vi "fom_parser.vi"(1 "fom_path (in)":path=path "C:/data/projects/730 - Engineering Laboratory/04 - Smart Grid/HLA Based Code Autogeneration/support/fom_examples/FedManager.xml", 5 "error in (no error)":errorcluster) -> (15 "interaction_descriptors (out)":T1[](array[typedef]), 19 "error out":errorcluster)   [LabVIEW 2016]
uses:
  pre-build/support/controls/raw_object_interaction_descriptor.ctl
  <vilib>/xml/Load XML File.vi
  <vilib>/xml/Close Reference(Node).vi
  <vilib>/xml/NI_XML.lvlib
  <resource>/objmgr/DOMUserDefRef.rc
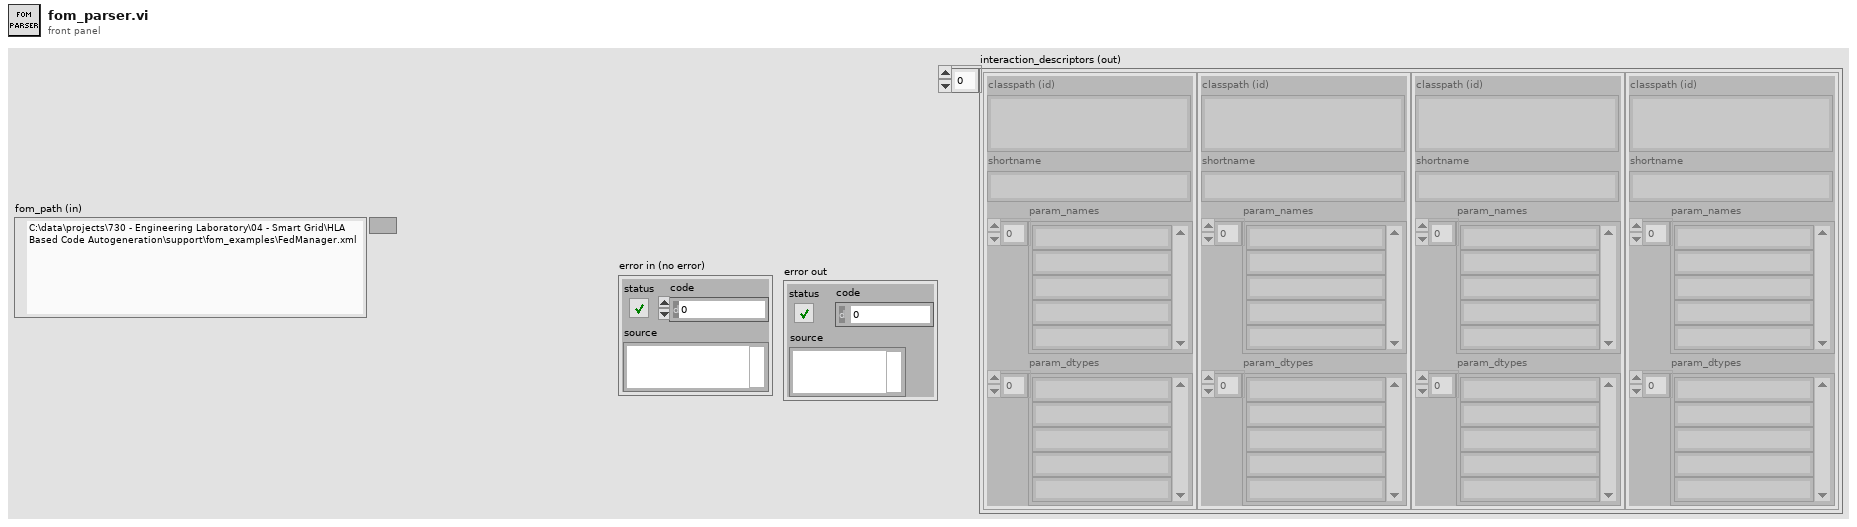
[diagram p1: front panel]
types:
  T1 = typedef "raw_object_interaction_descriptor.ctl" = cluster{"classpath (id)":string, "shortname":string, "param_names":string[], "param_dtypes":string[]}
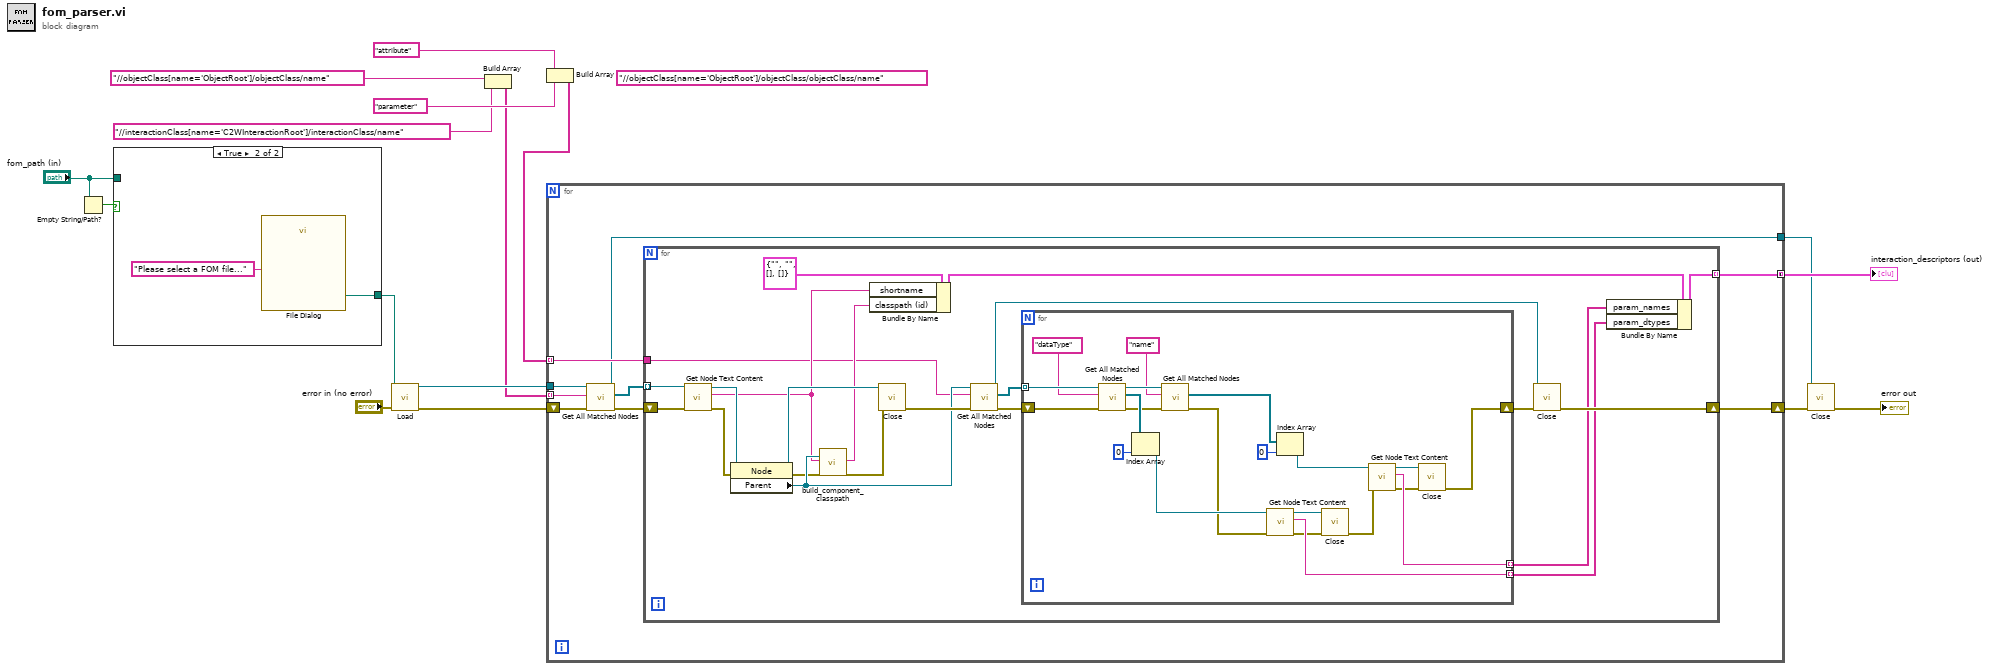
[diagram p0: block diagram]
diagram:
  (unwired) "//objectClass[name='ObjectRoot']/objectClass/objectClass/name"
  n1 = Empty String/Path?(string/path="fom_path (in)") -> (empty?=w12:bool)
  n2 = case shown="True" w12 {
    tunnel: [w17 w18] -> w10
    tunnel: "fom_path (in)" -> [w17 _]
    frame False {
    }
    frame True {
      n3 = call "File Dialog"("prompt"="Please select a FOM file...") -> ("selected path"=w18:path)  [unwired: 11 in, 3 out]
    }
  }
  n4 = call-poly <vilib>:"Load.vi"("path to XML document"=w10, "error in (no error)"="error in (no error)") -> ("DOM document out"=w16:refnum<k20>, "error out"=w15:errorcluster)  [unwired: 11 in, 1 out]
  n5 = Build Array("//objectClass[name='ObjectRoot']/objectClass/name", "//interactionClass[name='C2WInteractionRoot']/interactionClass/name") -> (w5:string[])
  n6 = Build Array("attribute", "parameter") -> (w4:string[])
  n7 = for {
    tunnel: w16 -> [w28]
    tunnel: [w24] -> w13 mode=concatenating
    tunnel: w5 -> [w23] mode=indexing
    shift-right: [w21] -> w3
    shift-left: w15 -> [w27]
    tunnel: w4 -> [w22] mode=indexing
    tunnel: [w20] -> w1
    n8 = call <vilib>:"Get All Matched Nodes.vi"("error in (no error)"=w27, "XPath expression"=w23, "node in"=w28) -> ("error out"=w25:errorcluster, "node result array"=w26:refnum<k20>[], "node out"=w20:refnum<k20>)  [unwired: 6 in]
    n9 = for {
      tunnel: w26 -> [w44] mode=indexing
      shift-right: [w47] -> w21
      shift-left: w25 -> [w45]
      tunnel: [w36] -> w24 mode=indexing
      tunnel: w22 -> [w29]
      n10 = call <vilib>:"Get Node Text Content.vi"("error in (no error)"=w45, "node in"=w44) -> ("error out"=w42:errorcluster, "node text"=w31:string, "node out"=w43:refnum<k20>)  [unwired: 7 in]
      n11 = property class="Node"(reference=w43, error in=w42) -> (reference out=w41:refnum<k20>, error out=w33:errorcluster, "Parent"=w34:refnum<k20>)
      n12 = call "build_component_classpath.vi"("1st_level_parent (in)"=w34, "comp_name (in)"=w31, "error in (no error)"=w33) -> ("classpath (out)"=w30:string, "error out"=w32:errorcluster)  [unwired: 15 in]
      n13 = Bundle By Name(cluster=T1 {"classpath (id)"="", "shortname"="", "param_names"=[], "param_dtypes"=[]} ("raw_info"), "shortname"=w31, "classpath (id)"=w30) -> (w35:T1)
      n14 = call-poly <vilib>:"Close.vi"("error in (no error)"=w32, "node"=w41) -> ("error out"=w40:errorcluster)  [unwired: 7 in]
      n15 = call <vilib>:"Get All Matched Nodes.vi"("error in (no error)"=w40, "XPath expression"=w29, "node in"=w34) -> ("error out"=w49:errorcluster, "node result array"=w50:refnum<k20>[], "node out"=w46:refnum<k20>)  [unwired: 6 in]
      n16 = for {
        tunnel: w50 -> [w67] mode=indexing
        tunnel: [w71] -> w38 mode=indexing
        shift-right: [w51] -> w48
        shift-left: w49 -> [w60]
        tunnel: [w63] -> w37 mode=indexing
        n17 = call <vilib>:"Get All Matched Nodes.vi"("error in (no error)"=w60, "XPath expression"="dataType", "node in"=w67) -> ("error out"=w61:errorcluster, "node result array"=w65:refnum<k20>[], "node out"=w62:refnum<k20>)  [unwired: 6 in]
        n18 = Index Array(array=w65, index=0) -> (element=w64:refnum<k20>)
        n19 = call <vilib>:"Get All Matched Nodes.vi"("error in (no error)"=w61, "XPath expression"="name", "node in"=w62) -> ("error out"=w57:errorcluster, "node result array"=w70:refnum<k20>[])  [unwired: 6 in, 1 out]
        n20 = call <vilib>:"Get Node Text Content.vi"("error in (no error)"=w57, "node in"=w64) -> ("error out"=w56:errorcluster, "node text"=w63:string, "node out"=w55:refnum<k20>)  [unwired: 7 in]
        n21 = Index Array(array=w70, index=0) -> (element=w68:refnum<k20>)
        n22 = call-poly <vilib>:"Close.vi"("error in (no error)"=w56, "node"=w55) -> ("error out"=w54:errorcluster)  [unwired: 7 in]
        n23 = call <vilib>:"Get Node Text Content.vi"("error in (no error)"=w54, "node in"=w68) -> ("error out"=w52:errorcluster, "node text"=w71:string, "node out"=w53:refnum<k20>)  [unwired: 7 in]
        n24 = call-poly <vilib>:"Close.vi"("error in (no error)"=w52, "node"=w53) -> ("error out"=w51:errorcluster)  [unwired: 7 in]
      }
      n25 = call-poly <vilib>:"Close.vi"("error in (no error)"=w48, "node"=w46) -> ("error out"=w47:errorcluster)  [unwired: 7 in]
      n26 = Bundle By Name(cluster=w35, "param_names"=w38, "param_dtypes"=w37) -> (w36:T1)
    }
  }
  "interaction_descriptors (out)" <- w13
  n27 = call-poly <vilib>:"Close.vi"("error in (no error)"=w3, "node"=w1) -> ("error out"=→"error out":errorcluster)  [unwired: 7 in]
